vi "Sans titre 2 (sous-VI).vi"(3 "Cc 2":dbl, 4 "T 2":dbl, 5 "Pièce 2":T1) -> (0 "Cc":dbl, 1 "T":dbl, 2 "Pièce":T1)   [LabVIEW 2010, in "lv_07.lvlib"]
uses:
  lv_07.lvlib
  c_pi_wilson.ctl
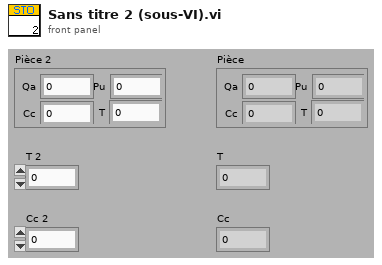
[diagram p1: front panel]
types:
  T1 = typedef "lv_07.lvlib/c_pi_wilson.ctl" = cluster{"T":dbl, "Pu":dbl, "Qa":dbl, "Cc":dbl}
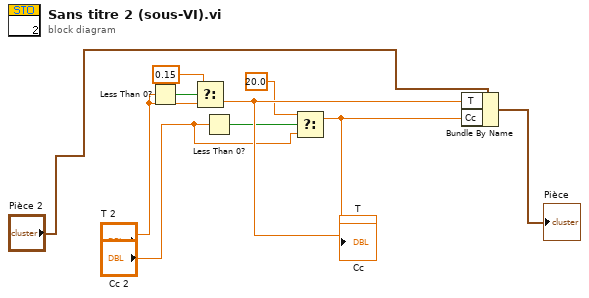
[diagram p0: block diagram]
diagram:
  n1 = Less Than 0?(x="T 2") -> (x < 0?=w1:bool)
  n2 = Select(t=0.15 ("cas vrai"), s=w1, f="T 2") -> (s? t:f=w8:dbl)
  "T" <- w8
  n3 = Less Than 0?(x="Cc 2") -> (x < 0?=w5:bool)
  n4 = Select(t=20.0 ("cas vrai"), s=w5, f="Cc 2") -> (s? t:f=w9:dbl)
  "Cc" <- w9
  n5 = Bundle By Name(cluster="Pièce 2", "T"=w8, "Cc"=w9) -> (→"Pièce":T1)
